vi "odczytaj_kursory.vi"(8 "error in (no error)":errorcluster, 11 "WaveformGraph in":refnum<vi>) -> (0 "error out":errorcluster, 4 "Array":string[][](array[string]))   [LabVIEW 2013]
doc: "Odczytuje wartoœci pozycji X i Y kursorów i wyœwietla do\nmultikolumn list box"
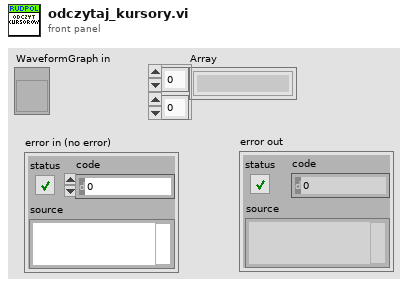
[diagram p1: front panel]
types:
  T1 = typedef "LVCursorListTypeDef.ctl" = cluster{"Name":string, "Color":u32, "Style":u8, "Point Style":u8, "Name Visible":bool, "Allow Drag":bool, "Cursor Mode":u32, "Plot":i32, "Index":i32, "Position":cluster{"X":dbl, "Y":dbl}, "X Scale":u32, "Y Scale":u32, "Watch Plots":i32[], "Watch All Plots":bool, "Plot Area":i32, "Label Offset":cluster{"X":dbl, "Y":dbl}}[]
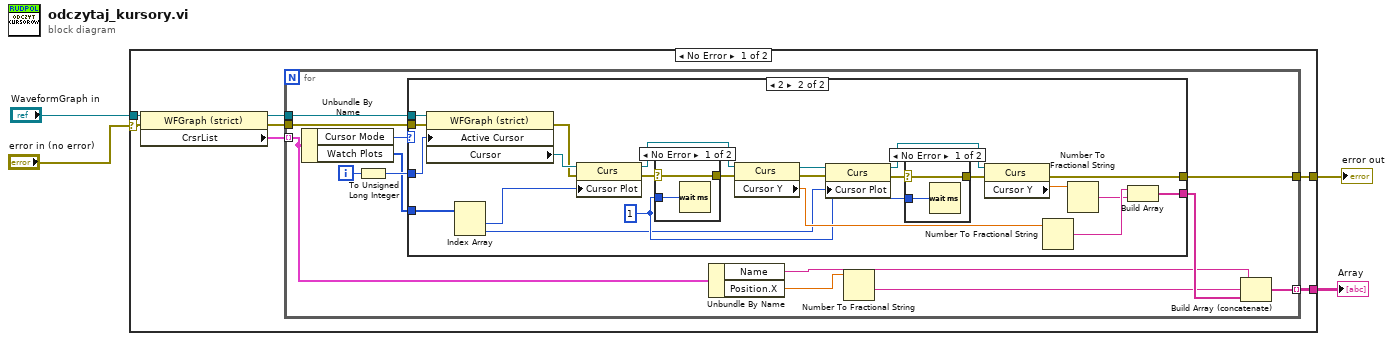
[diagram p0: block diagram]
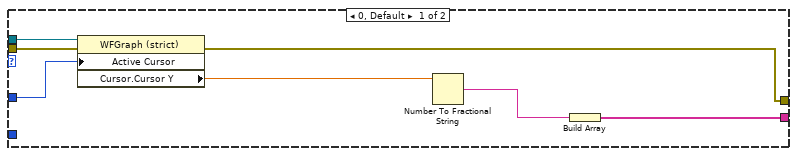
[diagram p2: hidden frame]
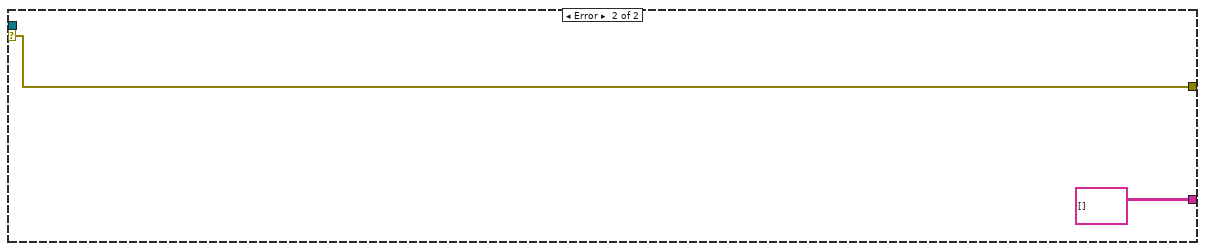
[diagram p5: hidden frame]
diagram:
  n1 = case shown="No Error" "error in (no error)" {
    selector: "error in (no error)" -> [w6 w62]
    tunnel: [w11 string[][] []] -> w4
    tunnel: "WaveformGraph in" -> [w8 _]
    tunnel: [w5 w62] -> w1
    frame No Error {
      n2 = property on="Property Node" class="WFGraph (strict)"(reference=w8, error in=w6) -> (reference out=w7:refnum<vi>, error out=w10:errorcluster, "CrsrList"=w9:T1)
      n3 = for {
        tunnel: w9 -> [w13] mode=indexing
        tunnel: w10 -> [w23]
        tunnel: [w20] -> w11 mode=indexing
        tunnel: w7 -> [w17]
        tunnel: [w16] -> w5
        i -> [w21]
        n4 = Unbundle By Name(w13) -> ("Cursor Mode"=w24:u32, "Watch Plots"=w14:i32[])
        n5 = To Unsigned Long Integer(number=w21) -> (unsigned 32bit integer=w22:u32)
        n6 = case shown="2" w24 {
          tunnel: w23 -> [w31 w52]
          tunnel: w22 -> [w30 w54]
          tunnel: [w27 w39] -> w19
          tunnel: w14 -> [_ w37]
          tunnel: w17 -> [w25 w34]
          tunnel: [w26 w32] -> w16
          frame 0, Default {
            n7 = property on="Property Node" class="WFGraph (strict)"(reference=w25, error in=w31, "Active Cursor"=w30) -> (error out=w26:errorcluster, "Cursor.Cursor Y"=w29:dbl)  [unwired: 1 out]
            n8 = Number To Fractional String(number=w29) -> (F-format string=w28:string)  [unwired: 3 in]
            n9 = Build Array(w28) -> (w27:string[])
          }
          frame 2 {
            w38 = u32 1 ("milliseconds to wait")
            n10 = property on="Property Node" class="WFGraph (strict)"(reference=w34, error in=w52, "Active Cursor"=w54) -> (error out=w33:errorcluster, "Cursor"=w53:refnum<vi>)  [unwired: 1 out]
            n11 = Index Array(array=w37) -> (element #1=w36:i32, element #2=w35:i32)  [unwired: 2 in]
            n12 = property class="Curs"(reference=w53, error in=w33, "Cursor Plot"=w36) -> (reference out=w50:refnum<vi>, error out=w51:errorcluster)
            n13 = case shown="No Error" w51 {
              selector: w51 -> [w59 w60]
              tunnel: [w59 w60] -> w49
              tunnel: w38 -> [w58 _]
              frame No Error {
                n14 = Wait (ms)(milliseconds to wait=w58) -> ()  [unwired: 1 out]
              }
              frame Error {
              }
            }
            n15 = property class="Curs"(reference=w50, error in=w49) -> (reference out=w45:refnum<vi>, error out=w44:errorcluster, "Cursor Y"=w42:dbl)
            n16 = property class="Curs"(reference=w45, error in=w44, "Cursor Plot"=w35) -> (reference out=w47:refnum<vi>, error out=w46:errorcluster)
            n17 = case shown="No Error" w46 {
              selector: w46 -> [w56 w57]
              tunnel: [w56 w57] -> w48
              tunnel: w38 -> [w55 _]
              frame No Error {
                n18 = Wait (ms)(milliseconds to wait=w55) -> ()  [unwired: 1 out]
              }
              frame Error {
              }
            }
            n19 = property class="Curs"(reference=w47, error in=w48) -> (error out=w32:errorcluster, "Cursor Y"=w43:dbl)  [unwired: 1 out]
            n20 = Number To Fractional String(number=w42) -> (F-format string=w41:string)  [unwired: 3 in]
            n21 = Number To Fractional String(number=w43) -> (F-format string=w40:string)  [unwired: 3 in]
            n22 = Build Array(w41, w40) -> (w39:string[])
          }
        }
        n23 = Unbundle By Name(w13) -> ("Name"=w12:string, "Position.X"=w15:dbl)
        n24 = Number To Fractional String(number=w15) -> (F-format string=w18:string)  [unwired: 3 in]
        n25 = Build Array (concatenate)(w12, w18, w19) -> (w20:string[])
      }
    }
    frame Error {
    }
  }
  "Array" <- w4
  "error out" <- w1
